vi "LC2-to-newtons.vi"(11 "mv in":dbl) -> (3 "newtons out":dbl)   [LabVIEW 2025]
uses:
  <vilib>/express/express arith-compare/Formula/XNode/ExpressFormulaBlockNode.xnode
  <vilib>/ptbypt/NI_PtbyPt.lvlib
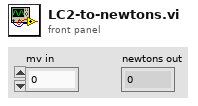
[diagram p1: front panel]
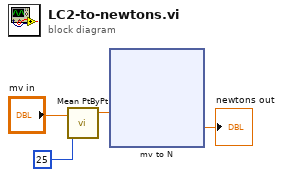
[diagram p0: block diagram]
diagram:
  n1 = call <vilib>:"Mean PtByPt.vi"("x"="mv in", "sample length"=25) -> ("mean"=w2:dbl)  [unwired: 2 in, 1 out]
  n2 = xnode ("mv to N")("mv"=w2) -> ("Result"=→"newtons out":dbl)  [unwired: 1 in, 1 out]
